vi "openbci_leadoff_impedance.vi"(4 "Test Signal N? (F)":bool, 6 "Test Signal P? (F)":bool, 8 "error in (no error)":errorcluster, 10 "channel":T3, 11 "OBCI dev in":T1={"COM port"="", "n_ch (8)"=enum."8 Channels", "delay_tx"=50}) -> (0 "error out":errorcluster, 3 "OBCI dev out":T1={"COM port"="", "n_ch (8)"=enum."8 Channels", "delay_tx"=50})   [LabVIEW 2013]
doc: "Set the Impedance testing for a specific channel (1 - 16)"
uses:
  Control Def/channels_enum.ctl
  Control Def/openbci_device.ctl
  Control Def/channel_count.ctl
  Control Def/string_channel_id.ctl
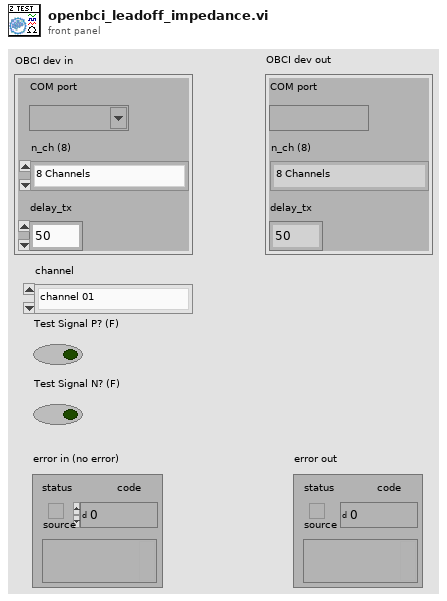
[diagram p1: front panel]
types:
  T1 = typedef "openbci_device.ctl" = cluster{"COM port":refnum<visa-resource-name>, "n_ch (8)":T2, "delay_tx":u32}
  T2 = typedef "channel_count.ctl" = enum16{"8 Channels", "16 Channels"}
  T3 = typedef "channels_enum.ctl" = enum16{"channel 01", "channel 02", "channel 03", "channel 04", "channel 05", "channel 06", "channel 07", "channel 08", "Channel 09", "Channel 10", "Channel 11", "Channel 12", "Channel 13", "Channel 14", "Channel 15", "Channel 16"}
  T4 = typedef "string_channel_id.ctl" = string[]
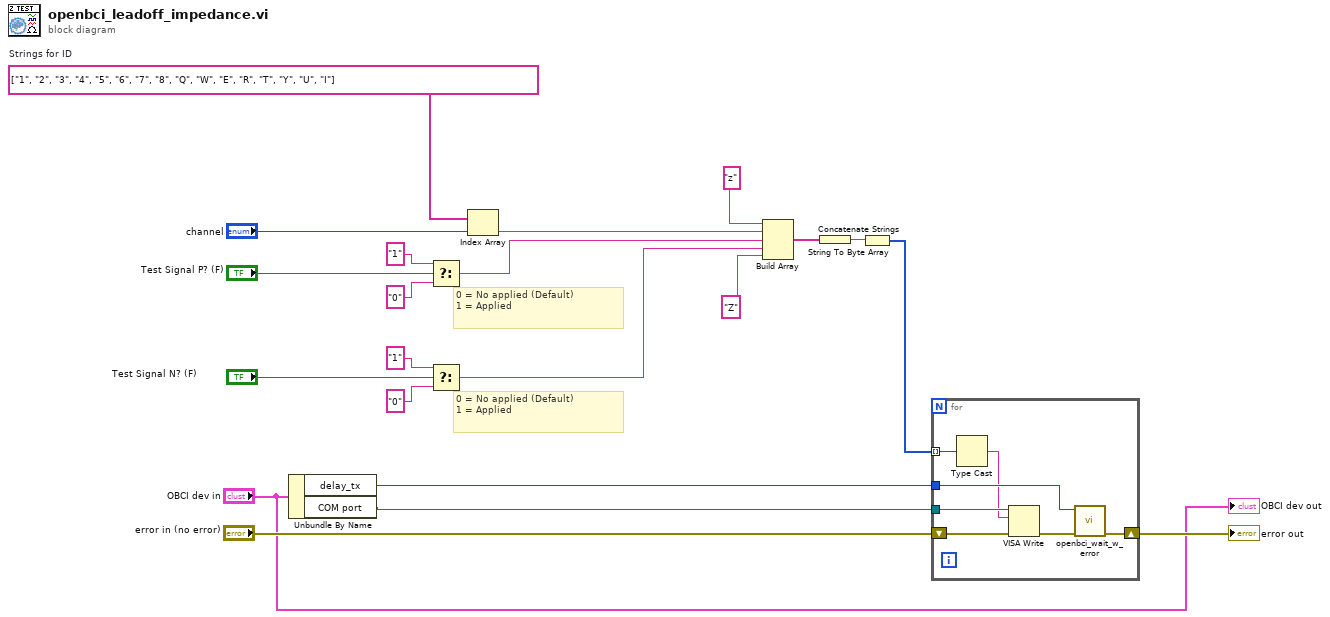
[diagram p0: block diagram]
diagram:
  w15 = T4 ["1", "2", "3", "4", "5", "6", "7", "8", "Q", "W", "E", "R", "T", "Y", "U", "I"]  # Strings for ID
  # "0 = No applied (Default)\n1 = Applied"
  # "0 = No applied (Default)\n1 = Applied"
  n1 = Unbundle By Name("OBCI dev in") -> ("delay_tx"=w17:u32, "COM port"=w19:refnum<visa-resource-name>)
  n2 = Select(t="1" ("element"), s="Test Signal P? (F)", f="0" ("element")) -> (s? t:f=w10:string)
  n3 = Select(t="1" ("element"), s="Test Signal N? (F)", f="0" ("element")) -> (s? t:f=w2:string)
  n4 = Index Array(array=w15, index="channel") -> (element=w14:string)
  n5 = Build Array("z" ("element"), w14, w10, w2, "Z" ("element")) -> (w7:string[])
  n6 = Concatenate Strings(w7) -> (w6:string)
  n7 = String To Byte Array(string=w6) -> (unsigned byte array=w5:u8[])
  n8 = for {
    tunnel: w19 -> [w27]
    tunnel: w17 -> [w24]
    tunnel: w5 -> [w22] mode=indexing
    shift-right: [w25] -> w18
    shift-left: "error in (no error)" -> [w28]
    n9 = Type Cast(x=w22) -> (*(type *) &x=w23:string)  [unwired: 1 in]
    n10 = VISA Write(VISA resource name=w27, write buffer=w23, error in (no error)=w28) -> (error out=w26:errorcluster)  [unwired: 2 out]
    n11 = call "openbci_wait_w_error.vi"("error in (no error)"=w26, "milliseconds to wait"=w24) -> ("error out"=w25:errorcluster)  [unwired: 9 in]
  }
  "error out" <- w18
  "OBCI dev out" <- "OBCI dev in"
